vi "Picture_Accquire.vi"(8 "Input Cluster 2":T6, 11 "Accquire":bool) -> (0 "output cluster":T6, 3 "New Value":bool)   [LabVIEW 2009]
uses:
  atmcd32d.llb/AcquisitionMode_mode typedef.ctl
  atmcd32d.llb/ReadMode_mode typedef.ctl
  atmcd32d.llb/TriggerMode_mode typedef.ctl
  atmcd32d.llb/Shutter_type typedef.ctl
  atmcd32d.llb/Shutter_mode typedef.ctl
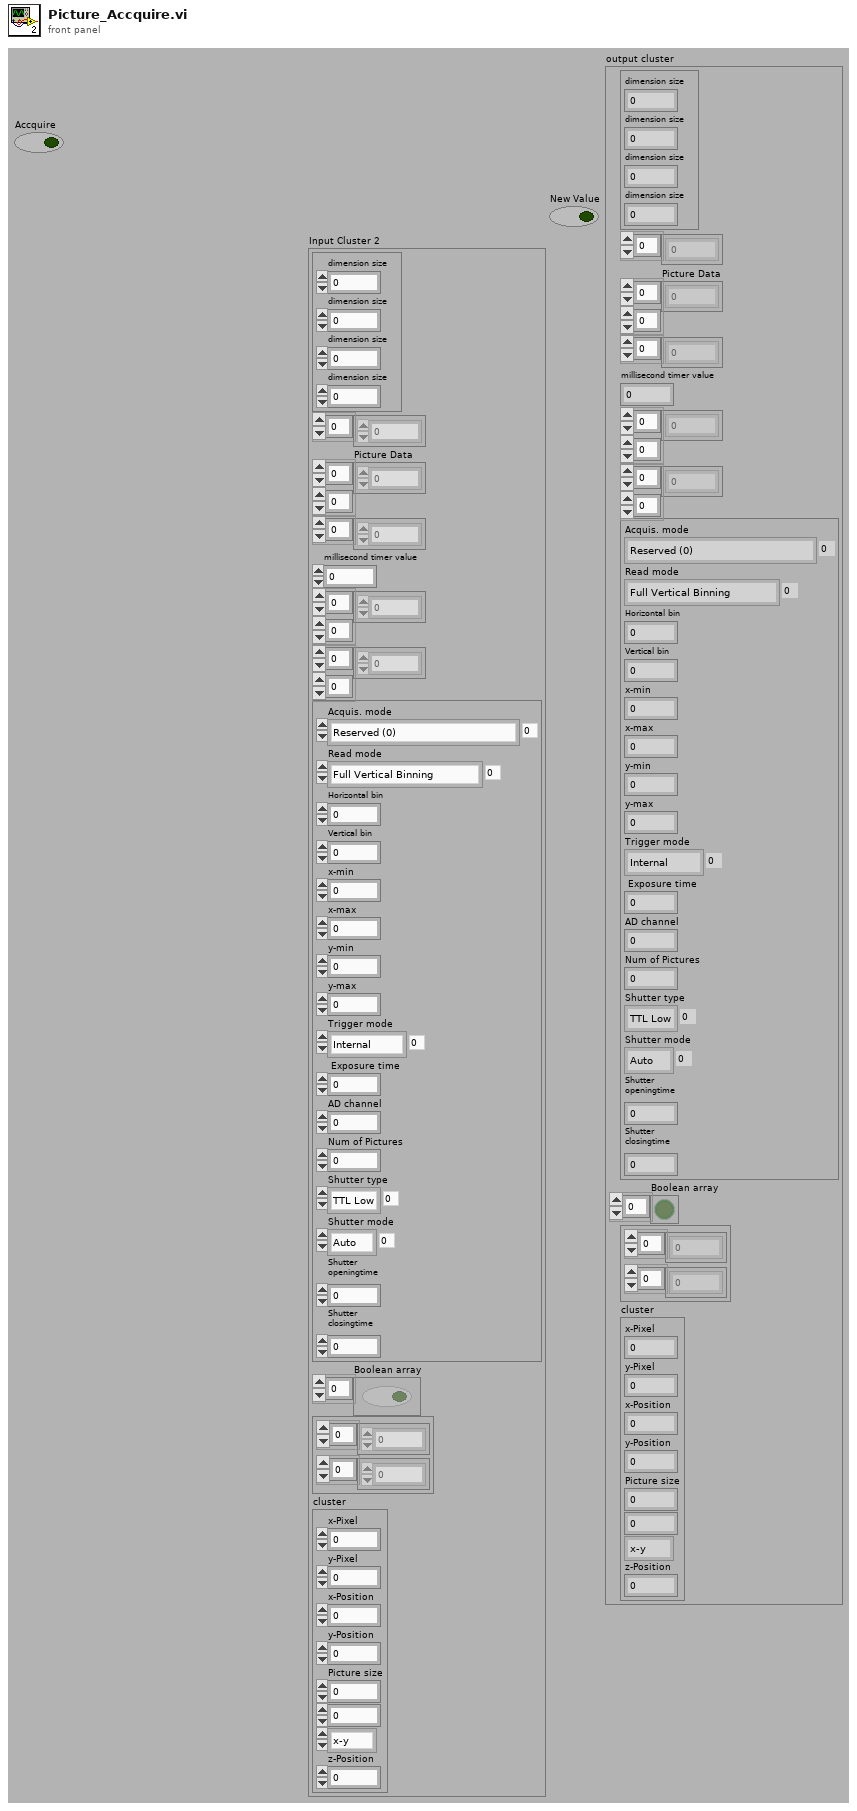
[diagram p1: front panel]
types:
  T1 = typedef "AcquisitionMode_mode typedef.ctl" = enum16{"Reserved (0)", "Single Scan", "Accumulate", "Kinetics", "Fast Kinetics", "Run Till Abort", "Reserved (6)", "Reserved (7)", "Reserved (8)", "Time Delayed Integration"}
  T2 = typedef "ReadMode_mode typedef.ctl" = enum16{"Full Vertical Binning", "Multi-Track", "Random-Track", "Single-Track", "Image"}
  T3 = typedef "TriggerMode_mode typedef.ctl" = enum16{"Internal", "External", "N/A (2)", "N/A (3)", "N/A (4)", "N/A (5)", "External Start"}
  T4 = typedef "Shutter_type typedef.ctl" = enum16{"TTL Low", "TTL High"}
  T5 = typedef "Shutter_mode typedef.ctl" = enum16{"Auto", "Open", "Close"}
  T6 = cluster{cluster{"dimension size":i32, "dimension size":i32, "dimension size":i32, "dimension size":i32}, i32[], "Picture Data":dbl[][], u32[], "millisecond timer value":u32, dbl[][], i32[][], cluster{"Acquis. mode":T1, "Read mode":T2, "Horizontal bin":i32, "Vertical bin":i32, "x-min":i32, "x-max":i32, "y-min":i32, "y-max":i32, "Trigger mode":T3, " Exposure time":sgl, "AD channel":i32, "Num of Pictures":i32, "Shutter type":T4, "Shutter mode":T5, "Shutter\nopeningtime":i32, "Shutter\nclosingtime":i32}, "Boolean array":bool[], cluster{dbl[], dbl[]}, "cluster":cluster{"x-Pixel":u16, "y-Pixel":u16, "x-Position":dbl, "y-Position":dbl, "Picture size":dbl, dbl, enum32{"x-y", "x-z", "y-z"}, "z-Position":dbl}}
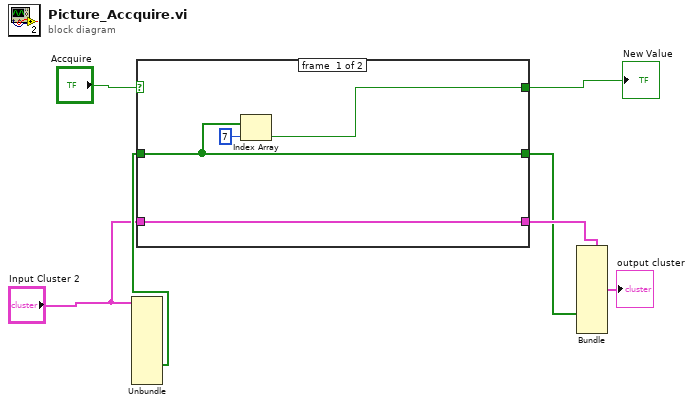
[diagram p0: block diagram]
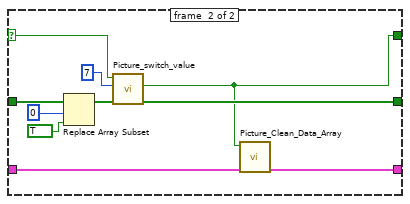
[diagram p2: hidden frame]
diagram:
  n1 = Unbundle("Input Cluster 2") -> ("Boolean array"=w5:bool[])  [unwired: 10 out]
  n2 = case shown="True" "Accquire" {
    selector: "Accquire" -> [_ w15]
    tunnel: w5 -> [w10 w21]
    tunnel: [w10 w16] -> w3
    tunnel: [w8 w14] -> w7
    tunnel: "Input Cluster 2" -> [w11 w13]
    tunnel: [w11 w12] -> w4
    frame #0 {
      n3 = Index Array(array=w10, index=7) -> (element=w8:bool)
    }
    frame #1 {
      n4 = Replace Array Subset(array=w21, new element=TRUE ("y"), index=0) -> (w17:bool[])
      n5 = call "Picture_switch_value.vi"("Boolean array in"=w17, "Value to switch"=7 ("index"), "Switch"=w15) -> ("Boolean array out"=w16:bool[], "New Value"=w14:bool)  [unwired: 7 out]
      n6 = call "Picture_Clean_Data_Array.vi"("Input Cluster"=w13, "Boolean"=w14) -> ("output cluster"=w12:T6)  [unwired: 9 out]
    }
  }
  "New Value" <- w7
  n7 = Bundle(cluster=w4, "Boolean array"=w3) -> (→"output cluster":T6)  [unwired: 10 out]
